vi "Compile Routing Channels.vi"(6 "Get Channel Data Refnum":refnum<vi>, 8 "error in (no error)":errorcluster, 10 "Communication Configuration":T2, 11 "Device Ref in":T5 format="%.0x") -> (0 "error out":errorcluster, 1 "Compiled Connections Buffer":T1[](array[typedef]), 2 "Routing Channels Configuration":T3[](array[typedef]), 3 "Device Ref out":T5 format="%.0x")   [LabVIEW 2020, in "Routing and Faulting System Explorer.lvlib"]
uses:
  Routing and Faulting System Explorer.lvlib
  <vilib>/NI VeriStand/Custom Device API/Custom Device Item Ref.ctl
  Shared/Routing Channel Configuration.ctl
  Shared/Value-Connections Map.ctl
  Shared/Communication Configuration.ctl
  Shared/Compiled Connection.ctl
  Shared/Routing and Faulting Shared.lvlib
  Scripting/Routing and Faulting Scripting.lvlib
  <vilib>/NI VeriStand/Custom Device API/Custom Device API.lvlib
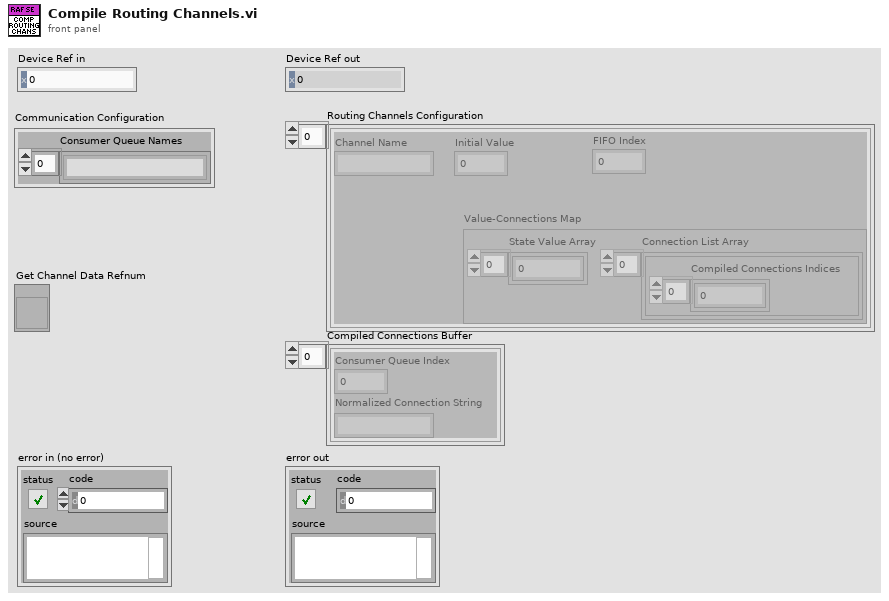
[diagram p1: front panel]
types:
  T1 = typedef "Routing and Faulting Shared.lvlib/Compiled Connection.ctl" = cluster{"Consumer Queue Index":i32, "Normalized Connection String":string}
  T2 = typedef "Routing and Faulting Shared.lvlib/Communication Configuration.ctl" = cluster{"Consumer Queue Names":string[]}
  T3 = typedef "Routing and Faulting Shared.lvlib/Routing Channel Configuration.ctl" = cluster{"Channel Name":string, "Initial Value":dbl, "FIFO Index":i32, "Value-Connections Map":T4}
  T4 = typedef "Routing and Faulting Shared.lvlib/Value-Connections Map.ctl" = cluster{"State Value Array":i32[], "Connection List Array":cluster{"Compiled Connections Indices":i32[]}[]}
  T5 = typedef "Custom Device API.lvlib/Custom Device Item Ref.ctl" = u64
  T6 = typedef "Routing and Faulting Shared.lvlib/Channel States.ctl" = T7[]
  T7 = typedef "Routing and Faulting Shared.lvlib/Routing State.ctl" = cluster{"Name":string, "Description":string, "Value":i32, "Connection List":T8[]}
  T8 = typedef "Routing and Faulting Shared.lvlib/Connection.ctl" = cluster{"Module":string, "Source":string, "Destination":string}
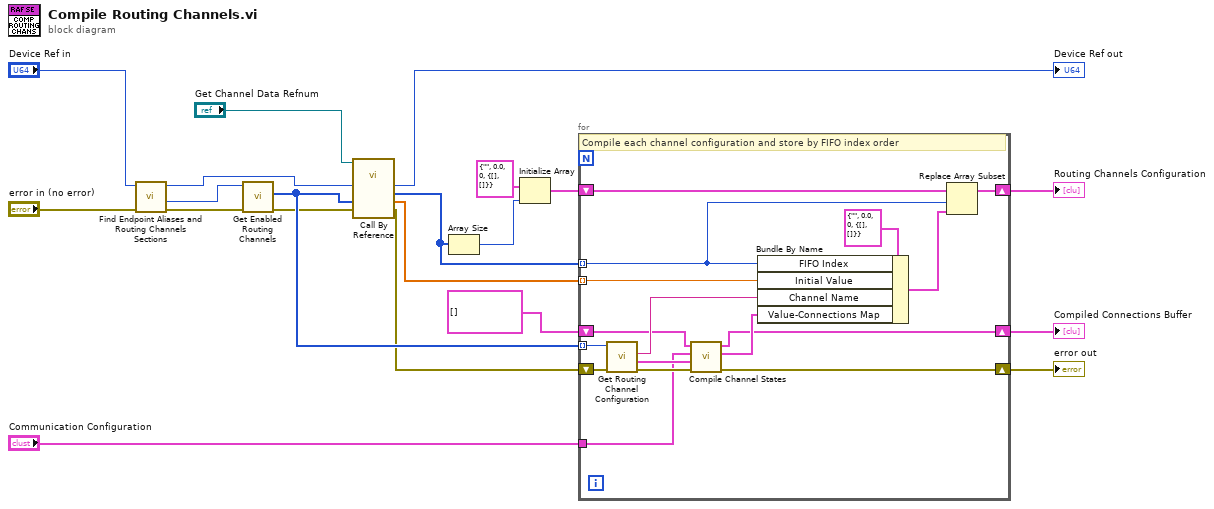
[diagram p0: block diagram]
diagram:
  n1 = call "Find Endpoint Aliases and Routing Channels Sections.vi"("error in"="error in (no error)", "routing and faulting custom device in"="Device Ref in") -> ("error out"=w2:errorcluster, "routing channels"=w1:T5, "routing and faulting custom device out"=w3:T5)  [unwired: 6 in, 1 out]
  n2 = call "Get Enabled Routing Channels.vi"("error in (no error)"=w2, "Routing Channels Ref in"=w1) -> ("error out"=w19:errorcluster, "Routing Channel Refs"=w20:T5[])  [unwired: 7 in, 1 out]
  n3 = call-by-ref "?"(reference="Get Channel Data Refnum", "error in (no error)"=w19, "Channel IDs"=w20, "Device Ref in"=w3) -> ("error out"=w18:errorcluster, "Default Values"=w17:dbl[], "FIFO Indices"=w15:i32[], "Device Ref out"=→"Device Ref out":T5)  [unwired: 5 in, 3 out]
  n4 = Array Size(array=w15) -> (size(s)=w14:i32)
  n5 = Initialize Array(T3 {"Channel Name"="", "Initial Value"=0.0, "FIFO Index"=0, "Value-Connections Map"={"State Value Array"=[], "Connection List Array"=[]}} ("Routing Channel Configuration"), w14) -> (w13:T3[])
  n6 = for {
    tunnel: w20 -> [w36] mode=indexing
    tunnel: w17 -> [w32] mode=indexing
    tunnel: w15 -> [w28] mode=indexing
    shift-right: [w30] -> w7
    shift-left: w18 -> [w33]
    shift-right: [w26] -> w12
    shift-left: w13 -> [w29]
    shift-right: [w21] -> w6
    shift-left: T1[] [] -> [w22]
    tunnel: "Communication Configuration" -> [w23]
    # "Compile each channel configuration and store by FIFO index order"
    n7 = call "Get Routing Channel Configuration.vi"("error in"=w33, "routing channel in"=w36) -> ("error out"=w31:errorcluster, "state configurations"=w24:T6, "routing channel name"=w34:string)  [unwired: 4 in, 3 out]
    n8 = call "Compile Channel States.vi"("error in (no error)"=w31, "Channel States"=w24, "Communication Configuration"=w23, "Compiled Connections Buffer in"=w22) -> ("error out"=w30:errorcluster, "Value-Connections Map"=w25:T4, "Compiled Connections Buffer out"=w21:T1[])  [unwired: 5 in]
    n9 = Bundle By Name(cluster=T3 {"Channel Name"="", "Initial Value"=0.0, "FIFO Index"=0, "Value-Connections Map"={"State Value Array"=[], "Connection List Array"=[]}} ("Routing Channel Configuration"), "FIFO Index"=w28, "Initial Value"=w32, "Channel Name"=w34, "Value-Connections Map"=w25) -> (w27:T3)
    n10 = Replace Array Subset(array=w29, new element=w27, index=w28) -> (w26:T3[])
  }
  "error out" <- w7
  "Routing Channels Configuration" <- w12
  "Compiled Connections Buffer" <- w6
